vi "Do.vi"(8 "error in (no error)":errorcluster, 10 "Actor in":refnum<class "Actor.lvclass">, 11 "Set Ratio Msg":refnum<class "Set Ratio Msg.lvclass">) -> (0 "error out":errorcluster, 2 "Actor out":refnum<class "Actor.lvclass">)   [LabVIEW 2020, in "BNT_ULx.lvlib" / "Set Ratio Msg.lvclass"]
doc: "This VI delivers the message to the actor by calling the appropriate method(s) on the actor."
uses:
  Set Ratio Msg.lvclass
  <vilib>/ActorFramework/Actor/Actor.lvclass
  C:/User/Brand/LVP/CSPP/CSPP-Template/Packages/CSPP_Core/Messages/CSPP_PVUpdate Msg/CSPP_PVUpdate Msg.lvclass
  CSPP_Core/Messages/CSPP_PVUpdate Msg/CSPP_PVUpdate Msg.lvclass/CSPP_PVUpdate Msg.ctl
  CSPP_Core/Classes/CSPP_ProcessVariables/ProcessVariable/PV.lvclass/PV.ctl
  Set Ratio Msg.lvclass/Set Ratio Msg.ctl
  CSPP_Core/Classes/CSPP_ProcessVariables/ProcessVariable/PV.lvclass
  <vilib>/regexp/Match Regular Expression.xnode
  CSPP_Core/Messages/CSPP_PVUpdate Msg/CSPP_PVUpdate Msg.lvclass
  BNT_ULx-MCSV-DOPWM/BNT_ULx-MCSV-DOPWM.lvclass
  C:/User/Brand/LVP/CSPP/CSPP-Template/Packages/CSPP_Core/Messages/CSPP_AsyncCallbackMsg/CSPP_AsyncCallback Msg.lvclass
  C:/Program Files (x86)/National Instruments/LabVIEW 2020/vi.lib/ActorFramework/Message/Message.lvclass
  C:/User/Brand/LVP/CSPP/CSPP-Template/Packages/BNT_ULx/BNT_ULx-MCSV/BNT_ULx-MCSV-DOPWM Messages/Set Ratio Msg/Set Ratio Msg.lvclass
  C:/User/Brand/LVP/CSPP/CSPP-Template/Packages/BNT_ULx/BNT_ULx-MCSV/BNT_ULx-MCSV/BNT_ULx-MCSV.lvclass
  C:/User/Brand/LVP/CSPP/CSPP-Template/Packages/CSPP_Core/Actors/CSPP_DeviceActor/CSPP_DeviceActor.lvclass
  C:/User/Brand/LVP/CSPP/CSPP-Template/Packages/CSPP_Core/Actors/CSPP_BaseActor/CSPP_BaseActor.lvclass
  C:/Program Files (x86)/National Instruments/LabVIEW 2020/vi.lib/ActorFramework/Actor/Actor.lvclass
  C:/User/Brand/LVP/CSPP/CSPP-Template/Packages/BNT_ULx/BNT_ULx-MCSV/BNT_ULx-MCSV-DOPWM/BNT_ULx-MCSV-DOPWM.lvclass
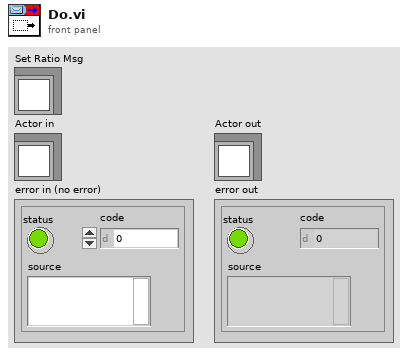
[diagram p1: front panel]
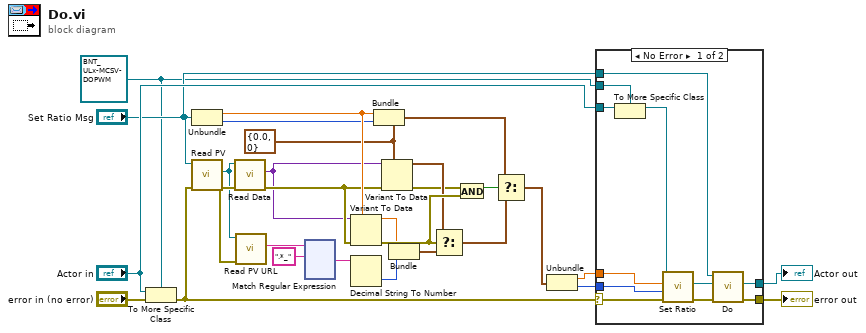
[diagram p0: block diagram]
diagram:
  w1 = refnum<class "BNT_ULx-MCSV-DOPWM.lvclass"> refnum ("BNT_ULx.lvlib:BNT_ULx-MCSV-DOPWM.lvclass")
  w7 = cluster{"Enable Channel":dbl, "Channel":i32} {"Enable Channel"=0.0, "Channel"=0} ("Type")
  n1 = To More Specific Class(target class=w1, reference="Actor in", error in="error in (no error)") -> (error out=w4:errorcluster)  [unwired: 1 out]
  n2 = Unbundle ("Pre-Unbundler")("Set Ratio Msg") -> (w18:dbl, w8:i32)
  n3 = call "Read PV.vi"("error in (no error)"=w4, "CS++PVUpdate Msg in"="Set Ratio Msg") -> ("error out"=w15:errorcluster, "PV"=w14:refnum<class "PV.lvclass">)  [unwired: 7 in, 1 out]
  n4 = call "Read Data.vi"("error in (no error)"=w15, "PV in"=w14) -> ("error out"=w17:errorcluster, "Data"=w16:variant)  [unwired: 7 in, 1 out]
  n5 = call "Read PV URL.vi"("error in (no error)"=w15, "PV in"=w14) -> ("PV URL"=w9:string)  [unwired: 7 in, 2 out]
  n6 = xnode "Match Regular Expression"("input string"=w9, "regular expression"=".*_") -> ("after match"=w11:string)  [unwired: 4 in, 4 out]
  n7 = Variant To Data(error in=w17, type=w18, Variant=w16) -> (data=w19:dbl, error out=w23:errorcluster)
  n8 = Decimal String To Number(string=w11) -> (number=w12:i32)  [unwired: 2 in, 1 out]
  n9 = Bundle ("Pre-Bundler")(cluster=w7, "Enable Channel"=w18, "Channel"=w8) -> (w6:cluster{"Enable Channel":dbl, "Channel":i32})
  n10 = Variant To Data(error in=w17, type=w7, Variant=w16) -> (data=w20:cluster{"Enable Channel":dbl, "Channel":i32}, error out=w5:errorcluster)
  n11 = Bundle ("Pre-Bundler")("PWM Ratio"=w19, w12) -> (w13:cluster{"PWM Ratio":dbl, i32})  [unwired: 1 in]
  n12 = Select ("MainSelect")(t=w20, s=w23, f=w13) -> (s? t:f=w21:cluster{"PWM Ratio":dbl, "Channel":i32})
  n13 = And(x=w5, y=w23) -> (x .and. y?=w22:bool)
  n14 = Select ("MainSelect")(t=w6, s=w22, f=w21) -> (s? t:f=w2:cluster{"PWM Ratio":dbl, "Channel":i32})
  n15 = Unbundle ("Main-Unbundler")(w2) -> ("PWM Ratio"=w25:dbl, "Channel"=w24:i32)
  n16 = case shown="No Error" w4 {
    selector: w4 -> [w31 w42]
    tunnel: [w37 w42] -> w28
    tunnel: [w38 w41] -> w27
    tunnel: "Actor in" -> [w40 w41]
    tunnel: w1 -> [w39 _]
    tunnel: "Set Ratio Msg" -> [w36 _]
    tunnel: w25 -> [w33 _]
    tunnel: w24 -> [w32 _]
    frame No Error {
      n17 = To More Specific Class ("To More Specific Class (internal)")(target class=w39, reference=w40) -> (specific class reference=w35:refnum<class "BNT_ULx-MCSV-DOPWM.lvclass">)  [unwired: 1 in, 1 out]
      n18 = call "Set Ratio.vi"("error in"=w31, "Line"=w32, "PWM Ratio"=w33, "BNT_ULx-MCSV-DOPWM in"=w35) -> ("error out"=w30:errorcluster, "BNT_ULx-MCSV-DOPWM out"=w34:refnum<class "BNT_ULx-MCSV-DOPWM.lvclass">)  [unwired: 6 in]
      n19 = call-parent "Do.vi"("error in (no error)"=w30, "Actor in"=w34, "CS++PVUpdate Msg"=w36) -> ("error out"=w37:errorcluster, "Actor out"=w38:refnum<class "Actor.lvclass">)  [unwired: 7 in]
    }
    frame Error {
    }
  }
  "error out" <- w28
  "Actor out" <- w27
